vi "Start.vi"(8 "error in (no error)":errorcluster, 10 "Params":variant, 11 "PmuAnalysis in":refnum<class "PmuAnalysis.lvclass">) -> (0 "error out":errorcluster, 3 "PmuAnalysis out":refnum<class "PmuAnalysis.lvclass">)   [LabVIEW 2018, in "AnalysisPlugins.lvlib" / "PmuAnalysis.lvclass"]
uses:
  PmuAnalysis.lvclass
  C:/projects/ICDAS/NistPluggableModules/Analysis/AnalysisPlugins/AnalysisPluginBaseClass/AnalysisPluginsBase.lvclass
  FGen/MemberClasses/PmuTestFunctions/Typedefs/PmuTestParams.ctl
  PmuAnalysis.lvclass/PmuAnalysis.ctl
  FGen/MemberClasses/PmuTestFunctions/Typedefs/eParamIdx.ctl
  AnalysisPluginBaseClass/AnalysisPluginsBase.lvclass/AnalysisPluginsBase.ctl
  Accessors/Read eTestType.vi
  AnalysisPluginBaseClass/Accessors/Write FileName.vi
  <vilib>/Utility/error.llb/Error Cluster From Error Code.vi
  FitterBaseClass/FitterBase.lvclass
  <vilib>/ErrorRing/Error Ring.xnode
  FGen/MemberClasses/PmuTestFunctions/PmuTestFunctions.lvclass
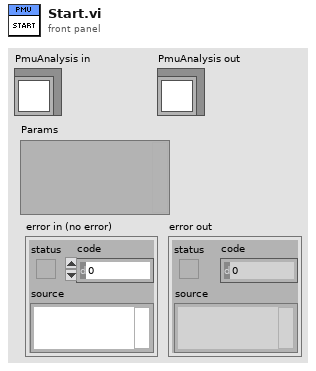
[diagram p1: front panel]
types:
  T1 = typedef "Functions.lvlib/PmuTestFunctions.lvclass/PmuTestParams.ctl" = dbl[][]
  T2 = typedef "Functions.lvlib/PmuTestFunctions.lvclass/eParamIdx.ctl" = enum16{"Xm", "Fin", "Ps", "Fh", "Ph", "Kh", "Fa", "Ka", "Fx", "Kx", "Rf", "KaS", "KxS", "KfS", "KrS"}
  T3 = enum16{"SteadyState", "Modulation", "Ramp", "Step"}
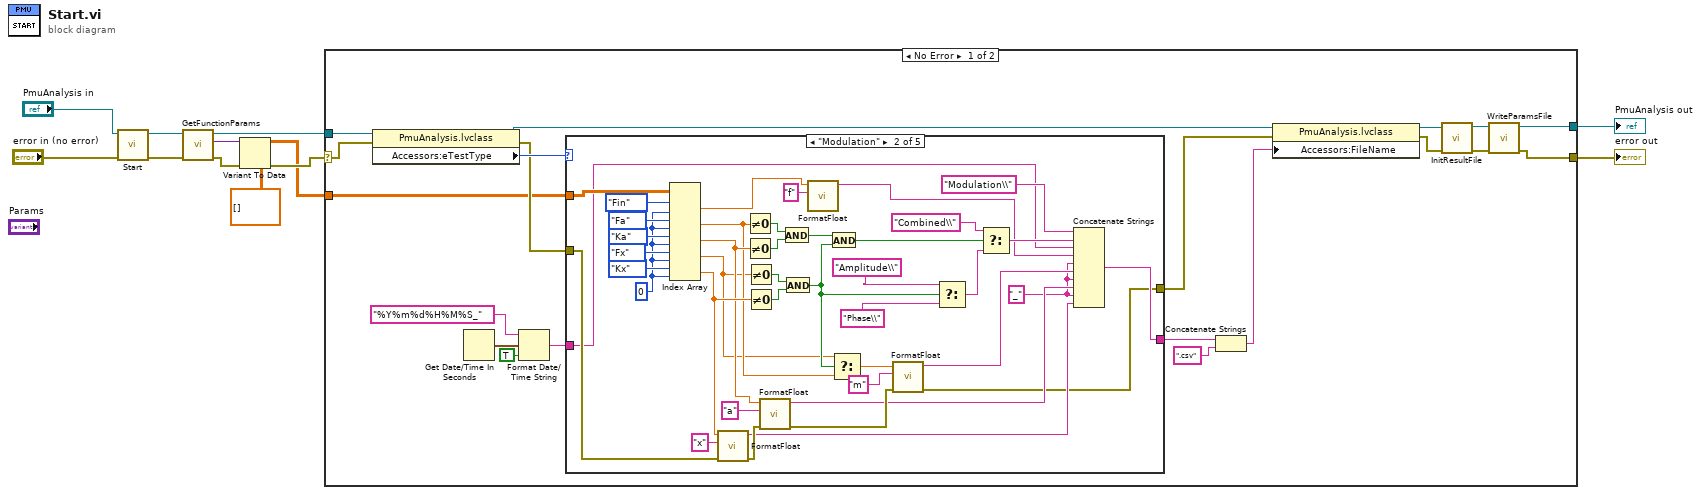
[diagram p0: block diagram]
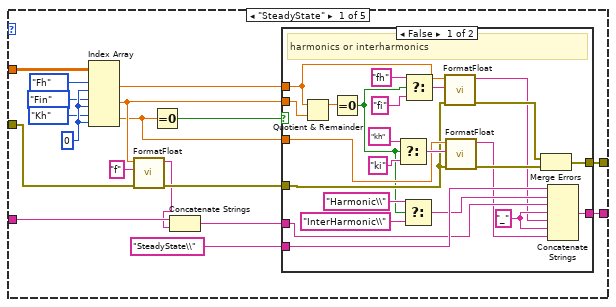
[diagram p2: hidden frame]
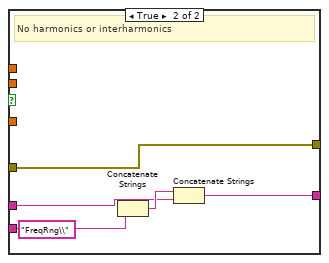
[diagram p3: hidden frame]
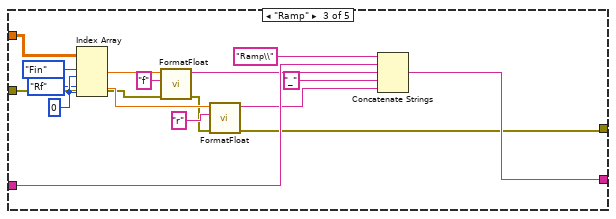
[diagram p4: hidden frame]
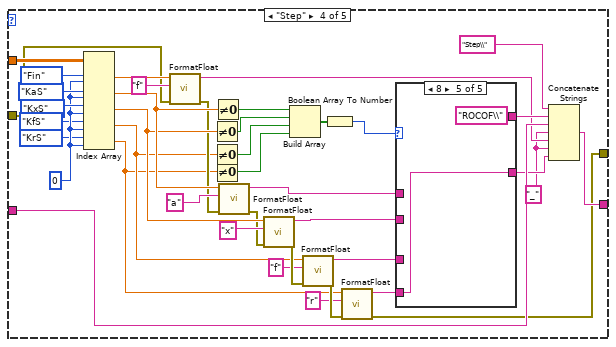
[diagram p5: hidden frame]
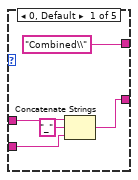
[diagram p6: hidden frame]
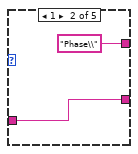
[diagram p7: hidden frame]
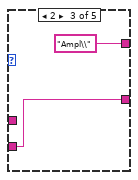
[diagram p8: hidden frame]
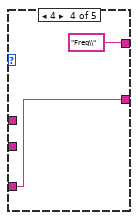
[diagram p9: hidden frame]
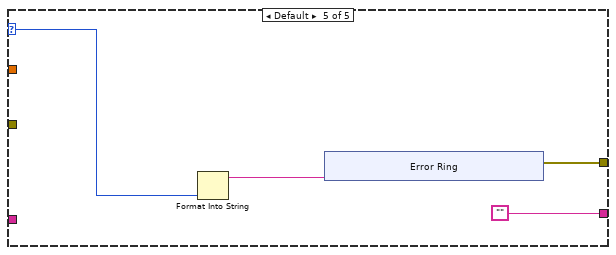
[diagram p10: hidden frame]
diagram:
  n1 = call-parent "Start.vi"("error in (no error)"="error in (no error)", "FitterBase in"="PmuAnalysis in") -> ("error out"=w7:errorcluster, "FitterBase out"=w8:refnum<class "PmuAnalysis.lvclass">)  [unwired: 8 in]
  n2 = call-dynamic "GetFunctionParams.vi"("error in (no error)"=w7, "PmuAnalysis in"=w8) -> ("error out"=w3:errorcluster, "FunctionParams"=w4:variant, "PmuAnalysis out"=w6:refnum<class "PmuAnalysis.lvclass">)  [unwired: 7 in]
  n3 = Variant To Data(error in=w3, type=T1 [] ("Accessors:PmuTestParams"), Variant=w4) -> (data=w1:T1, error out=w2:errorcluster)
  n4 = case shown="No Error" w2 {
    selector: w2 -> [w15 w203]
    tunnel: w6 -> [w16 w204]
    tunnel: [w18 w204] -> w10
    tunnel: [w17 w203] -> w9
    tunnel: w1 -> [w13 _]
    frame No Error {
      n5 = property class="PmuAnalysis.lvclass"(reference=w16, error in=w15) -> (reference out=w27:refnum<class "PmuAnalysis.lvclass">, error out=w14:errorcluster, "Accessors:eTestType"=w32:T3)
      n6 = Get Date/Time In Seconds() -> (seconds since 1Jan1904=w30:timestamp)
      n7 = Format Date/Time String(time format string (%c)="%Y%m%d%H%M%S_", seconds (now)=w30, UTC format=TRUE) -> (date/time string=w28:string)
      n8 = case shown="\"Modulation\"" w32 {
        selector: w32 -> [_ _ _ _ w194]
        tunnel: w14 -> [w45 w109 w130 w172 _]
        tunnel: w13 -> [w50 w121 w138 w178 _]
        tunnel: w28 -> [w41 w99 w127 w157 _]
        tunnel: [w34 w92 w123 w153 ""] -> w25
        tunnel: [w33 w91 w122 w139 w193] -> w24
        frame "SteadyState" {
          w48 = 0 ("disabled index (col)")
          n9 = Index Array(array=w50, index (row) #1=eParamIdx."Fh" ("eParamIdx"), index (col) #1=w48, index (row) #2=eParamIdx."Fin" ("eParamIdx"), index (col) #2=w48, index (row) #3=eParamIdx."Kh" ("eParamIdx"), index (col) #3=w48) -> (element #1=w37:dbl, element #2=w36:dbl, element #3=w35:dbl)
          n10 = call "FormatFloat.vi"("error in (no error)"=w45, "replace string (\".\")"="f" ("replace string (\".\")"), "float"=w36) -> ("error out"=w42:errorcluster, "string"=w40:string)  [unwired: 7 in]
          n11 = Equal To 0?(x=w35) -> (x = 0?=w43:bool)
          n12 = Concatenate Strings(w41, w40) -> (w39:string)
          n13 = case shown="False" w43 {
            tunnel: w42 -> [w60 w75]
            tunnel: w39 -> [w54 w77]
            tunnel: "SteadyState\\" -> [w59 w80]
            tunnel: [w67 w76] -> w34
            tunnel: [w73 w75] -> w33
            tunnel: w37 -> [w66 _]
            tunnel: w36 -> [w65 _]
            tunnel: w35 -> [w61 _]
            frame False {
              w52 = "_" ("string")
              # "harmonics or interharmonics"
              n14 = Quotient & Remainder(x=w66, y=w65) -> (x-y*floor(x/y)=w64:dbl)  [unwired: 1 out]
              n15 = Equal To 0?(x=w64) -> (x = 0?=w56:bool)
              n16 = Select(t="kh" ("replace string (\".\")"), s=w56, f="ki" ("replace string (\".\")")) -> (s? t:f=w70:string)
              n17 = Select(t="Harmonic\\", s=w56, f="InterHarmonic\\") -> (s? t:f=w55:string)
              n18 = Select(t="fh" ("replace string (\".\")"), s=w56, f="fi" ("replace string (\".\")")) -> (s? t:f=w74:string)
              n19 = call "FormatFloat.vi"("error in (no error)"=w60, "replace string (\".\")"=w74, "float"=w66) -> ("error out"=w72:errorcluster, "string"=w51:string)  [unwired: 7 in]
              n20 = call "FormatFloat.vi"("error in (no error)"=w60, "replace string (\".\")"=w70, "float"=w61) -> ("error out"=w71:errorcluster, "string"=w53:string)  [unwired: 7 in]
              n21 = Merge Errors(w72, w71) -> (w73:errorcluster)
              n22 = Concatenate Strings(w59, w55, w54, w52, w51, w52, w53) -> (w67:string)
            }
            frame True {
              # "No harmonics or interharmonics"
              n23 = Concatenate Strings(w80, "FreqRng\\") -> (w78:string)
              n24 = Concatenate Strings(w78, w77) -> (w76:string)
            }
          }
        }
        frame "Modulation" {
          w83 = "_" ("string")
          w90 = 0 ("disabled index (col)")
          n25 = Index Array(array=w121, index (row) #1=eParamIdx."Fin" ("eParamIdx"), index (col) #1=w90, index (row) #2=eParamIdx."Fa" ("eParamIdx"), index (col) #2=w90, index (row) #3=eParamIdx."Ka" ("eParamIdx"), index (col) #3=w90, index (row) #4=eParamIdx."Fx" ("eParamIdx"), index (col) #4=w90, index (row) #5=eParamIdx."Kx" ("eParamIdx"), index (col) #5=w90) -> (element #1=w86:dbl, element #2=w82:dbl, element #3=w88:dbl, element #4=w81:dbl, element #5=w110:dbl)
          n26 = call "FormatFloat.vi"("error in (no error)"=w109, "replace string (\".\")"="x" ("replace string (\".\")"), "float"=w110) -> ("error out"=w107:errorcluster, "string"=w93:string)  [unwired: 7 in]
          n27 = Not Equal To 0?(x=w82) -> (x != 0?=w115:bool)
          n28 = Not Equal To 0?(x=w88) -> (x != 0?=w116:bool)
          n29 = Not Equal To 0?(x=w81) -> (x != 0?=w114:bool)
          n30 = Not Equal To 0?(x=w110) -> (x != 0?=w113:bool)
          n31 = call "FormatFloat.vi"("error in (no error)"=w107, "replace string (\".\")"="a" ("replace string (\".\")"), "float"=w88) -> ("error out"=w95:errorcluster, "string"=w94:string)  [unwired: 7 in]
          n32 = And(x=w115, y=w116) -> (x .and. y?=w112:bool)
          n33 = And(x=w114, y=w113) -> (x .and. y?=w98:bool)
          n34 = call "FormatFloat.vi"("replace string (\".\")"="f" ("replace string (\".\")"), "float"=w86) -> ("string"=w84:string)  [unwired: 8 in, 1 out]
          n35 = And(x=w112, y=w98) -> (x .and. y?=w106:bool)
          n36 = Select(t=w81, s=w98, f=w82) -> (s? t:f=w97:dbl)
          n37 = call "FormatFloat.vi"("error in (no error)"=w95, "replace string (\".\")"="m" ("replace string (\".\")"), "float"=w97) -> ("error out"=w91:errorcluster, "string"=w85:string)  [unwired: 7 in]
          n38 = Select(t="Amplitude\\", s=w98, f="Phase\\") -> (s? t:f=w102:string)
          n39 = Select(t="Combined\\", s=w106, f=w102) -> (s? t:f=w100:string)
          n40 = Concatenate Strings("Modulation\\", w100, w99, w84, w83, w85, w83, w94, w83, w93) -> (w92:string)
        }
        frame "Ramp" {
          w137 = 0 ("disabled index (col)")
          n41 = Index Array(array=w138, index (row) #1=eParamIdx."Fin" ("eParamIdx"), index (col) #1=w137, index (row) #2=eParamIdx."Rf" ("eParamIdx"), index (col) #2=w137) -> (element #1=w134:dbl, element #2=w132:dbl)
          n42 = call "FormatFloat.vi"("error in (no error)"=w130, "replace string (\".\")"="f" ("replace string (\".\")"), "float"=w134) -> ("error out"=w129:errorcluster, "string"=w126:string)  [unwired: 7 in]
          n43 = call "FormatFloat.vi"("error in (no error)"=w129, "replace string (\".\")"="r" ("replace string (\".\")"), "float"=w132) -> ("error out"=w122:errorcluster, "string"=w124:string)  [unwired: 7 in]
          n44 = Concatenate Strings("Ramp\\" ("string"), w127, w126, "_" ("string"), w124) -> (w123:string)
        }
        frame "Step" {
          w154 = "_" ("string")
          w152 = 0 ("disabled index (col)")
          n45 = Index Array(array=w178, index (row) #1=eParamIdx."Fin" ("eParamIdx"), index (col) #1=w152, index (row) #2=eParamIdx."KaS" ("eParamIdx"), index (col) #2=w152, index (row) #3=eParamIdx."KxS" ("eParamIdx"), index (col) #3=w152, index (row) #4=eParamIdx."KfS" ("eParamIdx"), index (col) #4=w152, index (row) #5=eParamIdx."KrS" ("eParamIdx"), index (col) #5=w152) -> (element #1=w174:dbl, element #2=w171:dbl, element #3=w170:dbl, element #4=w145:dbl, element #5=w144:dbl)
          n46 = call "FormatFloat.vi"("error in (no error)"=w172, "replace string (\".\")"="f" ("replace string (\".\")"), "float"=w174) -> ("error out"=w167:errorcluster, "string"=w156:string)  [unwired: 7 in]
          n47 = Not Equal To 0?(x=w170) -> (x != 0?=w164:bool)
          n48 = Not Equal To 0?(x=w145) -> (x != 0?=w149:bool)
          n49 = Not Equal To 0?(x=w144) -> (x != 0?=w148:bool)
          n50 = Not Equal To 0?(x=w171) -> (x != 0?=w165:bool)
          n51 = call "FormatFloat.vi"("error in (no error)"=w167, "replace string (\".\")"="a" ("replace string (\".\")"), "float"=w171) -> ("error out"=w166:errorcluster, "string"=w161:string)  [unwired: 7 in]
          n52 = call "FormatFloat.vi"("error in (no error)"=w166, "replace string (\".\")"="x" ("replace string (\".\")"), "float"=w170) -> ("error out"=w147:errorcluster, "string"=w160:string)  [unwired: 7 in]
          n53 = Build Array(w165, w164, w149, w148) -> (w163:bool[])
          n54 = call "FormatFloat.vi"("error in (no error)"=w147, "replace string (\".\")"="f" ("replace string (\".\")"), "float"=w145) -> ("error out"=w146:errorcluster, "string"=w141:string)  [unwired: 7 in]
          n55 = Boolean Array To Number(Boolean array=w163) -> (number=w162:u32)
          n56 = call "FormatFloat.vi"("error in (no error)"=w146, "replace string (\".\")"="r" ("replace string (\".\")"), "float"=w144) -> ("error out"=w139:errorcluster, "string"=w140:string)  [unwired: 7 in]
          n57 = case shown="8" w162 {
            tunnel: ["Combined\\" "Phase\\" "Ampl\\" "Freq\\" "ROCOF\\"] -> w159
            tunnel: [w182 w184 w186 w188 w190] -> w155
            tunnel: w161 -> [w181 w184 _ _ _]
            tunnel: w160 -> [w179 _ w186 _ _]
            tunnel: w141 -> [_ _ _ w188 _]
            tunnel: w140 -> [_ _ _ _ w190]
            frame 0, Default {
              n58 = Concatenate Strings(w181, "_" ("string"), w179) -> (w182:string)
            }
            frame 1 {
            }
            frame 2 {
            }
            frame 4 {
            }
            frame 8 {
            }
          }
          n59 = Concatenate Strings("Step\\", w159, w157, w154, w156, w154, w155) -> (w153:string)
        }
        frame Default {
          n60 = Format Into String(w194) -> (resulting string=w195:string)  [unwired: 3 in, 1 out]
          n61 = xnode "Error Ring"("parameter 0"=w195) -> ("error out"=w193:errorcluster)
        }
      }
      n62 = Concatenate Strings(w25, ".csv" ("string")) -> (w23:string)
      n63 = property class="PmuAnalysis.lvclass"(reference=w27, error in=w24, "Accessors:FileName"=w23) -> (reference out=w22:refnum<class "PmuAnalysis.lvclass">, error out=w21:errorcluster)
      n64 = call-dynamic "InitResultFile.vi"("error in (no error)"=w21, "PmuAnalysis in"=w22) -> ("error out"=w20:errorcluster, "PmuAnalysis out"=w19:refnum<class "PmuAnalysis.lvclass">)  [unwired: 8 in]
      n65 = call "WriteParamsFile.vi"("error in (no error)"=w20, ":PmuAnalysis"=w19) -> ("error out"=w17:errorcluster, "PmuAnalysis"=w18:refnum<class "PmuAnalysis.lvclass">)  [unwired: 8 in]
    }
    frame Error {
    }
  }
  "error out" <- w9
  "PmuAnalysis out" <- w10
